vi "_emi_ SMLoop Restart.vi"(0 "Loop Index/Numb":u16, 1 "Action(Get Index)":T2=enum."Get index", 7 "Value":T1) -> (4 "Index out":u16, 8 "Value out":T1, 10 "Size":i32)   [LabVIEW 2011]
uses:
  Loop control/Private/_emi_Loop control int action.ctl
  _emi_ SMLoop restart type.ctl
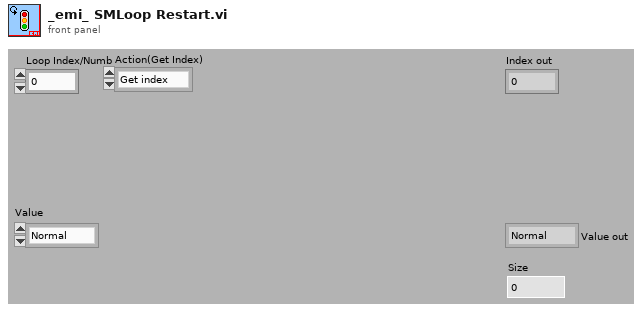
[diagram p1: front panel]
types:
  T1 = typedef "_emi_ SMLoop restart type.ctl" = enum16{"Normal", "Stop", "Stopped"}
  T2 = typedef "_emi_Loop control int action.ctl" = enum16{"Init index", "Get index", "Set index", "Get Size"}
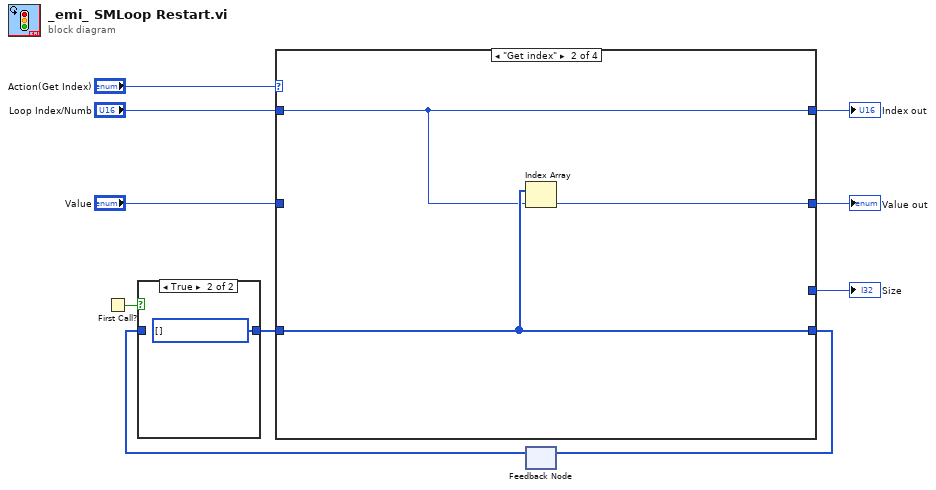
[diagram p0: block diagram]
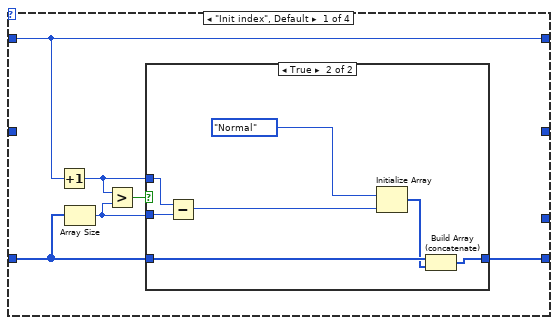
[diagram p2: hidden frame]
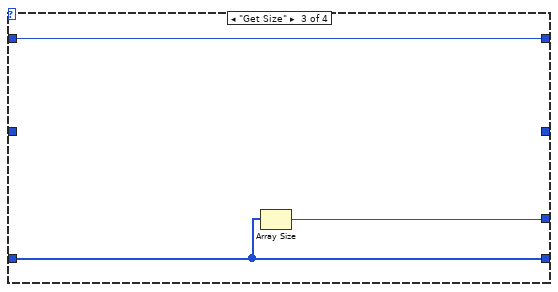
[diagram p4: hidden frame]
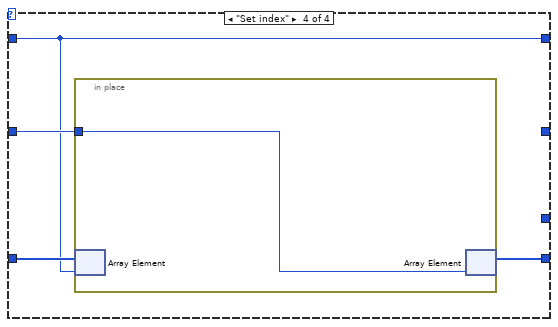
[diagram p5: hidden frame]
diagram:
  n1 = First Call?() -> (First Call?: T/F=w10:bool)
  n2 = feedback #1() -> (w4:T1[])  [unwired: 1 in]
  n3 = case shown="True" w10 {
    tunnel: [w11 w12] -> w5
    tunnel: w4 -> [w11 _]
    frame False {
    }
    frame True {
      w12 = T1[] [] items=["Normal", "Stop", "Stopped"]
    }
  }
  n4 = case shown="\"Get index\"" "Action(Get Index)" {
    tunnel: [w18 w28 w32 w33] -> w9
    tunnel: "Loop Index/Numb" -> [w18 w28 w32 w33]
    tunnel: [w14 w29 w31 w35] -> w6
    tunnel: w5 -> [w13 w29 w31 w36]
    tunnel: [_ w27 _ _] -> w1
    tunnel: "Value" -> [_ _ _ w34]
    tunnel: [_ _ w30 _] -> w3
    frame "Init index", Default {
      n5 = Increment(x=w18) -> (x+1=w15:u16)
      n6 = Array Size(array=w13) -> (size(s)=w16:i32)
      n7 = Greater?(x=w15, y=w16) -> (0:w17:bool)
      n8 = case shown="True" w17 {
        tunnel: w16 -> [_ w25]
        tunnel: w15 -> [_ w26]
        tunnel: [w19 w21] -> w14
        tunnel: w13 -> [w19 w23]
        frame False {
        }
        frame True {
          n9 = Subtract(x=w26, y=w25) -> (x-y=w24:i32)
          n10 = Initialize Array(_emi__SMLoop_restart_type."Normal" ("Value out"), w24) -> (w22:T1[])
          n11 = Build Array (concatenate)(w23, w22) -> (w21:T1[])
        }
      }
    }
    frame "Get index" {
      n12 = Index Array(array=w29, index=w28) -> (element=w27:T1)
    }
    frame "Get Size" {
      n13 = Array Size(array=w31) -> (size(s)=w30:i32)
    }
    frame "Set index" {
      n14 = in-place {
        in-place-border: w34 -> [w37]
        n15 = in-place-array #2(w36, w33) -> ()  [unwired: 1 out]
        n16 = in-place-array #2(w37) -> (w35:T1[])  [unwired: 1 out]
      }
    }
  }
  "Index out" <- w9
  "Size" <- w3
  "Value out" <- w1
  n17 = feedback-in #1(w6) -> ()
